vi "Get DataType+.vi"(8 "Error In":errorcluster, 11 "reference in":refnum<class "OD Entry.lvclass">) -> (0 "Error Out":errorcluster, 1 "Defined?":bool, 2 "DataType":T1 items=["UNKNOWN", "BOOLEAN", "INTEGER8", "INTEGER16", "INTEGER32", "UNSIGNED8", "UNSIGNED16", "UNSIGNED32", "REAL32", "VISIBLE_STRING", "OCTET_STRING", "UNICODE_STRING", "TIME_OF_DAY", "TIME_DIFFERENCE", "RESERVED1", "DOMAIN", "INTEGER24", "REAL64", "INTEGER40", "INTEGER48", "INTEGER56", "INTEGER64", "UNSIGNED24", "RESERVED2", "UNSIGNED40", "UNSIGNED48", "UNSIGNED56", "UNSIGNED64", "RESERVED3", "RESERVED4", "RESERVED5", "RESERVED6", "PDO_COMMUNICATION_PARAMETER", "PDO_MAPPING", "SDO_PARAMETER", "IDENTITY", "RESERVED7"], 3 "reference out":refnum<class "OD Entry.lvclass">)   [LabVIEW 2024, in "EDS.lvlib" / "OD Entry.lvclass"]
uses:
  OD Entry.lvclass
  OD Entry.lvclass/OD Entry.ctl
  Object Type/Object Type Base.lvclass
  Data Type.ctl
  EDS.lvlib
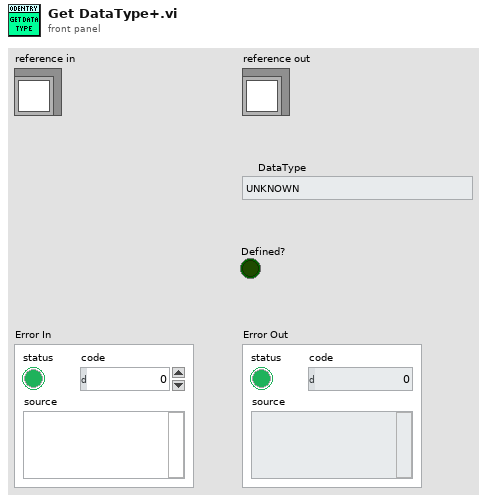
[diagram p1: front panel]
types:
  T1 = typedef "EDS.lvlib/Data Type.ctl" = u16
  T2 = typedef "EDS.lvlib/OD Entry.lvclass/ObjectAttributes.ctl" = cluster{"Index":u16, "ObjectType":refnum<class "Object Type Base.lvclass">, "Denotation":string, "Count":u8, "ObjExtend":u8, "PDOtype":T3, "Label":string, "Description":string, "Sub-Entries":map{u8, refnum<class "OD Sub-Entry.lvclass">}}
  T3 = typedef "EDS.lvlib/PDO Mapping Type.ctl" = enum16{"NO", "OPTIONAL", "RPDO", "TPDO", "DEFAULT"}
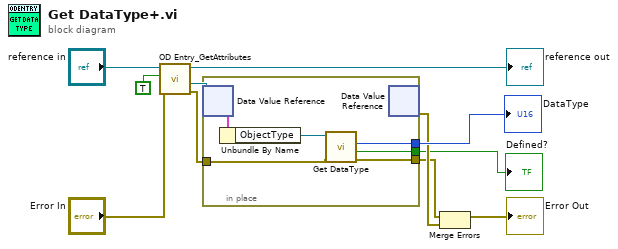
[diagram p0: block diagram]
diagram:
  n1 = call "OD Entry_GetAttributes.vi"("Error In"="Error In", "OnlyGetDvrReference(False)"=TRUE, "reference in"="reference in") -> ("Error Out"=w3:errorcluster, "DataRef"=w4:refnum<data-value>, "reference out"=→"reference out":refnum<class "OD Entry.lvclass">)  [unwired: 5 in, 1 out]
  n2 = in-place {
    in-place-border: [w15] -> w7
    in-place-border: w3 -> [w14]
    in-place-border: [w13] -> w2
    in-place-border: [w12] -> w1
    n3 = in-place-dvr #1(w4) -> (w16:T2)  [unwired: 1 out]
    n4 = Unbundle By Name(w16) -> ("ObjectType"=w17:refnum<class "Object Type Base.lvclass">)
    n5 = call-dynamic "Get DataType.vi"("error in"=w14, "Object Type in"=w17) -> ("error out"=w13:errorcluster, "Set?"=w12:bool, "DataType"=w15:T1)  [unwired: 6 in, 1 out]
    n6 = in-place-dvr #1() -> (w6:errorcluster)  [unwired: 1 in, 1 out]
  }
  "DataType" <- w7
  "Defined?" <- w1
  n7 = Merge Errors(w2, w6) -> (→"Error Out":errorcluster)
